vi "rs3 init disparity_to_depth.vi"(8 "error in (no error)":errorcluster) -> (0 "error out":errorcluster, 1 "error frame queue":u64, 2 "error disp transf block":u64, 3 "error start processing":u64, 4 "disparity_transforg_2_block":u64, 5 "disparity transforg_2_queue":u64)   [LabVIEW 2018, in "libRealSense3.lvlib"]
doc: "This initialized the processing block & queue to be able to transform from disparity space to depth (z=1/D)."
uses:
  libRealSense3.lvlib
  realsense2.dll
panel:
  # "RS3 Init Disparity-To-Depth"
  # "(C) Intel Corp.,  AGJ"
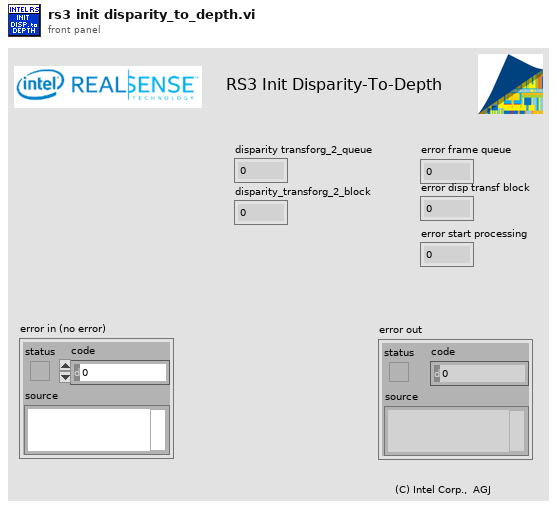
[diagram p1: front panel]
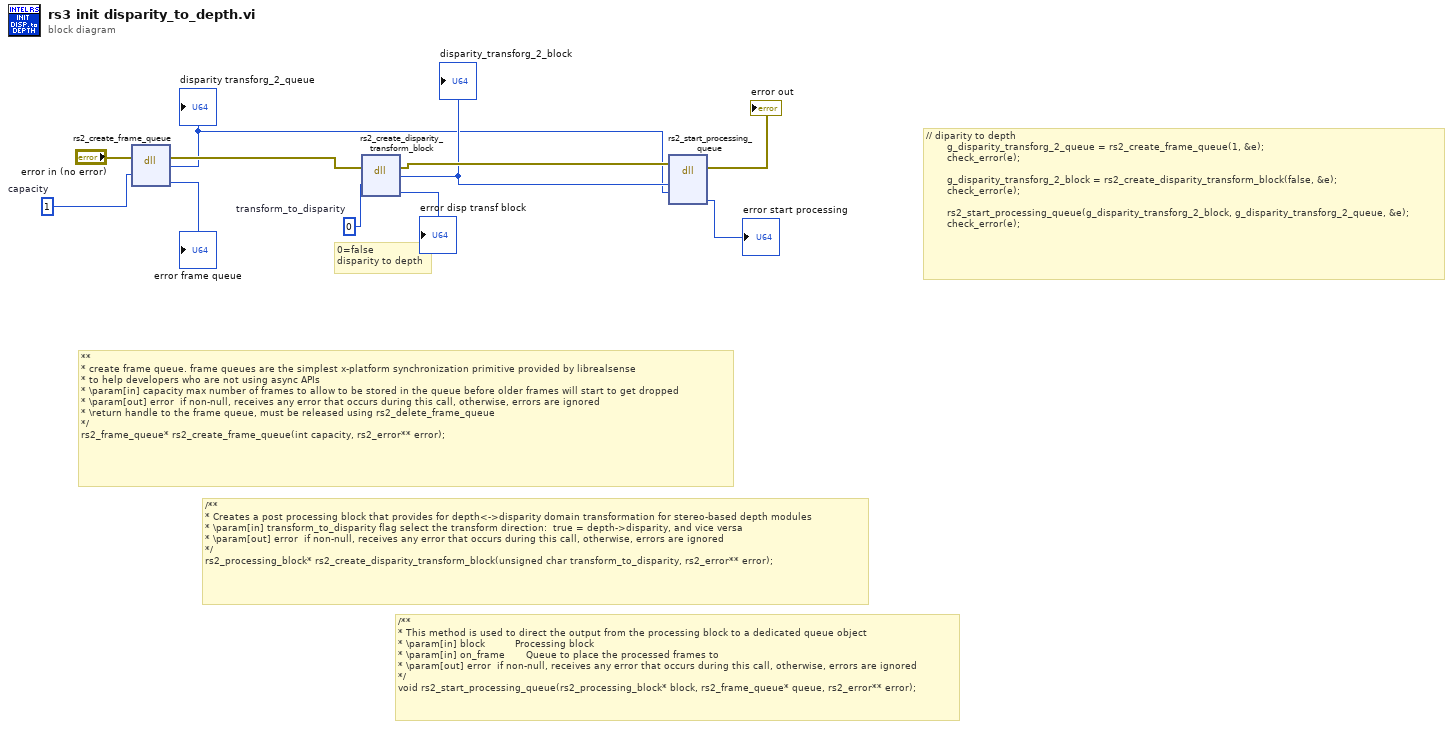
[diagram p0: block diagram]
diagram:
  w10 = 1  # capacity
  w1 = u8 0  # transform_to_disparity
  # "0=false \ndisparity to depth"
  # "/**\n* Creates a post processing block that provides for depth<->disparity domain transformation for stereo-based depth modules\n* \\param[in] transform_to_disparity flag select the transform direction:  true = depth->disparity, and vice versa\n* \\param[out] error  if non-null, receives any error that occurs during this call, otherwise, errors are ignored\n*/\nrs2_processing_block* rs2_create_disparity_transform_block(unsigned char transform_to_disparity, rs2_error** error);"
  # "// diparity to depth\n       g_disparity_transforg_2_queue = rs2_create_frame_queue(1, &e);\n       check_error(e);\n\n       g_disparity_transforg_2_block = rs2_create_disparity_transform_block(false, &e);\n       check_error(e);\n\n       rs2_start_processing_queue(g_disparity_transforg_2_block, g_disparity_transforg_2_queue, &e);\n       check_error(e);"
  # "/**\n* This method is used to direct the output from the processing block to a dedicated queue object\n* \\param[in] block          Processing block\n* \\param[in] on_frame       Queue to place the processed frames to\n* \\param[out] error  if non-null, receives any error that occurs during this call, otherwise, errors are ignored\n*/\nvoid rs2_start_processing_queue(rs2_processing_block* block, rs2_frame_queue* queue, rs2_error** error);"
  # "**\n* create frame queue. frame queues are the simplest x-platform synchronization primitive provided by librealsense\n* to help developers who are not using async APIs\n* \\param[in] capacity max number of frames to allow to be stored in the queue before older frames will start to get dropped\n* \\param[out] error  if non-null, receives any error that occurs during this call, otherwise, errors are ignored\n* \\return handle to the frame queue, must be released using rs2_delete_frame_queue\n*/\nrs2_frame_queue* rs2_create_frame_queue(int capacity, rs2_error** error);"
  n1 = dll-call lib="C:/Users/aaron.jencks/Documents/GitHub/emerson_seed_object_detection/LabVIEW/Projects/Paul's Video Viewer/Classes/Realsense Cam/realsense_wrapper_api/realsense2.dll" fn="rs2_create_frame_queue"(error in="error in (no error)", "capacity"=w10) -> (error out=w8:errorcluster, "decimation filter queue"=w3:u64, "error"=→"error frame queue":u64)  [unwired: 4 in, 1 out]
  "disparity transforg_2_queue" <- w3
  n2 = dll-call lib="C:/Users/aaron.jencks/Documents/GitHub/emerson_seed_object_detection/LabVIEW/Projects/Paul's Video Viewer/Classes/Realsense Cam/realsense_wrapper_api/realsense2.dll" fn="rs2_create_disparity_transform_block"(error in=w8, "transform_to_disparity"=w1) -> (error out=w6:errorcluster, "disparity_transform_1_block"=w4:u64, "error"=→"error disp transf block":u64)  [unwired: 4 in, 1 out]
  "disparity_transforg_2_block" <- w4
  n3 = dll-call lib="C:/Users/aaron.jencks/Documents/GitHub/emerson_seed_object_detection/LabVIEW/Projects/Paul's Video Viewer/Classes/Realsense Cam/realsense_wrapper_api/realsense2.dll" fn="rs2_start_processing_queue"(error in=w6, "processing block"=w4, "frame queue"=w3) -> (error out=→"error out":errorcluster, "error"=→"error start processing":u64)  [unwired: 6 in, 1 out]
